vi "UHR-Fleezers Control (host) - 12.2.vi"() -> ()   [LabVIEW 2012] (continued)
            n651 = Wait (ms)(milliseconds to wait=u32 250) -> ()  [unwired: 1 out]
          }
          frame #6 {
            n652 = property on="Start Saving" class="Bool (strict)"("Val(Sgnl)"=TRUE ("Value (Signaling)")) -> ()  [unwired: 2 in, 2 out]
            n653 = Wait (ms)(milliseconds to wait=u32 5000) -> ()  [unwired: 1 out]
          }
          frame #7 {
            w1054 = TRUE ("Value (Signaling)")
            n654 = property on="Rem fb disp offset" class="Bool (strict)"("Val(Sgnl)"=w1054) -> ()  [unwired: 2 in, 2 out]
            n655 = property on="Remove Offset" class="Bool (strict)"("Val(Sgnl)"=w1054) -> ()  [unwired: 2 in, 2 out]
            n656 = Wait (ms)(milliseconds to wait=u32 100) -> ()  [unwired: 1 out]
          }
          frame #8 {
            n657 = case shown="True" w1057 {
              frame False {
              }
              frame True {
                n658 = local write "Trap Trig. Fl."(TRUE ("Value (Signaling)")) -> ()
              }
            }
          }
          frame #9 {
            n659 = case shown="True" "Start dipping after?" {
              frame False {
              }
              frame True {
                n660 = flat-sequence {
                  frame #0 {
                    n661 = Multiply(x="Delay before dipping (s)", y=1000.0) -> (x*y=w1061:dbl)
                    n662 = Wait (ms)(milliseconds to wait=w1061) -> ()  [unwired: 1 out]
                  }
                  frame #1 {
                    n663 = property on="Dip for Protein" class="Bool (strict)"("Val(Sgnl)"=TRUE ("Value (Signaling)")) -> ()  [unwired: 2 in, 2 out]
                    n664 = local write "Scripts"(T1."Dipping" ("Scripts")) -> ()
                  }
                }
              }
            }
          }
        }
      }
      event "Fixed Traps Data\nScript": Value Change {
        n665 = event-data() -> ()  [unwired: 1 in, 5 out]
        n666 = flat-sequence {
          frame #0 {
            n667 = case shown="True" "Green ON" {
              frame False {
              }
              frame True {
                n668 = property on="Green Laser ON/Interlacing" class="Bool (strict)"("Val(Sgnl)"=TRUE) -> ()  [unwired: 2 in, 2 out]
              }
            }
            n669 = local write "Offset (nm)"(0.0 ("Offset (nm)")) -> ()
            n670 = property on="Sample Channel\nFlow" class="Bool (strict)"("Val(Sgnl)"=FALSE ("Value (Signaling)")) -> ()  [unwired: 2 in, 2 out]
            n671 = property on="Trap Delta (MHz)" class="DigNum (strict)"("Val(Sgnl)"="Fixed Traps Trap Delta (MHz)") -> ()  [unwired: 2 in, 2 out]
          }
          frame #1 {
            n672 = Wait (ms)(milliseconds to wait=u32 1000) -> ()  [unwired: 1 out]
          }
          frame #2 {
            n673 = local write "Start Saving"(TRUE ("Start Saving")) -> ()
          }
          frame #3 {
            n674 = local read "Bead Sep. Int. Time (s)"() -> (w1072:dbl)
            n675 = Multiply(x=w1072, y=1000.0) -> (x*y=w1074:dbl)
            n676 = Wait (ms)(milliseconds to wait=w1074) -> ()  [unwired: 1 out]
          }
          frame #4 {
            n677 = property on="Remove Offset" class="Bool (strict)"("Val(Sgnl)"=TRUE ("Value (Signaling)")) -> ()  [unwired: 2 in, 2 out]
          }
          frame #5 {
            n678 = property on="Dip for Protein" class="Bool (strict)"("Val(Sgnl)"="Start dipping after?") -> ()  [unwired: 2 in, 2 out]
          }
        }
      }
      event "Got DNA bead": Value Change {
        n679 = event-data() -> ()  [unwired: 1 in, 5 out]
        n680 = flat-sequence {
          frame #0 {
            n681 = local read "Daq spot flow on"() -> (w1079:bool)
            n682 = case shown="True" w1079 {
              frame False {
              }
              frame True {
                n683 = property on="Sample Channel\nFlow" class="Bool (strict)"("Val(Sgnl)"=TRUE ("Value (Signaling)")) -> ()  [unwired: 2 in, 2 out]
              }
            }
            n684 = property on="Got DNA bead" class="Bool"("Key Focus"=FALSE) -> ()  [unwired: 2 in, 2 out]
          }
          frame #1 {
            n685 = property on="Inject Pump 1" class="Bool (strict)"("Val(Sgnl)"=FALSE ("Value (Signaling)")) -> ()  [unwired: 2 in, 2 out]
          }
          frame #2 {
            n686 = property on="Cal/Data Acq. Spot" class="Bool (strict)"("Val(Sgnl)"=TRUE ("Value (Signaling)")) -> ()  [unwired: 2 in, 2 out]
          }
        }
      }
      event "Take Stepping Data": Value Change {
        n687 = event-data() -> ()  [unwired: 1 in, 5 out]
        n688 = local read "Save ave N"() -> (w1091:dbl)
        n689 = flat-sequence {
          tunnel: w1091 -> [w1093]
          tunnel: [w1093] -> w1086
          tunnel: [w1095] -> w1087
          tunnel: w1086 -> [w1095]
          tunnel: [w1097] -> w1088
          tunnel: w1087 -> [w1097]
          tunnel: [w1100] -> w1089
          tunnel: w1088 -> [w1100]
          tunnel: [w1102] -> w1090
          tunnel: w1089 -> [w1102]
          tunnel: [w1104] -> w1084
          tunnel: w1090 -> [w1104]
          tunnel: w1084 -> [w1107]
          tunnel: [w1107] -> w1083
          tunnel: w1083 -> [w1108]
          tunnel: [w1108] -> w1085
          tunnel: w1085 -> [w1114]
          frame #0 {
            n690 = property on="Save ave N" class="DigNum (strict)"("Val(Sgnl)"="Save ave factor") -> ()  [unwired: 2 in, 2 out]
          }
          frame #1 {
            n691 = Wait (ms)(milliseconds to wait=u32 100) -> ()  [unwired: 1 out]
          }
          frame #2 {
            n692 = local read "Offset 2 Start (MHz)"() -> (w1099:dbl)
            n693 = property on="Saved AOD Raster Scan Parameter Sets" class="Arr (strict)"("Index Values"=u32[] [2]) -> ()  [unwired: 2 in, 2 out]
            n694 = property on="Trap Delta (MHz)" class="DigNum (strict)"("Val(Sgnl)"=w1099) -> ()  [unwired: 2 in, 2 out]
          }
          frame #3 {
            n695 = property on="Load parameters" class="Bool (strict)"("Val(Sgnl)"=TRUE ("Value (Signaling)")) -> ()  [unwired: 2 in, 2 out]
          }
          frame #4 {
            n696 = Wait (ms)(milliseconds to wait=u32 100) -> ()  [unwired: 1 out]
          }
          frame #5 {
            n697 = property on="Trap Raster Scan" class="Bool (strict)"("Val(Sgnl)"=TRUE ("Value (Signaling)")) -> ()  [unwired: 2 in, 2 out]
          }
          frame #6 {
            n698 = Wait (ms)(milliseconds to wait=u32 1000) -> ()  [unwired: 1 out]
          }
          frame #7 {
            n699 = while {
              stop <- w1111 stop-if-true
              n700 = local read "Raster Scanning..."() -> (w1113:bool)
              n701 = local read "Saving..."() -> (w1112:bool)
              n702 = Not(x=w1112) -> (.not. x?=w1109:bool)
              n703 = Not(x=w1113) -> (.not. x?=w1110:bool)
              n704 = And(x=w1110, y=w1109) -> (x .and. y?=w1111:bool)
            }
          }
          frame #8 {
            n705 = property on="Save ave N" class="DigNum (strict)"("Val(Sgnl)"=w1114) -> ()  [unwired: 2 in, 2 out]
          }
        }
      }
      event "Step Size (nm)": Value Change {
        n706 = event-data() -> ()  [unwired: 1 in, 5 out]
        n707 = flat-sequence {
          frame #0 {
            n708 = property on="Saved AOD Raster Scan Parameter Sets" class="Arr (strict)"("Index Values"=u32[] [1]) -> ()  [unwired: 2 in, 2 out]
          }
          frame #1 {
            n709 = Multiply(x="N Steps", y="Step Size (nm)") -> (x*y=w1116:dbl)
            n710 = property on="Scan Speed AOD (nm/s) 2" class="DigNum (strict)"("Value"="Step Size (nm)") -> ()  [unwired: 2 in, 2 out]
            n711 = property on="Step Size AOD (nm) 2" class="DigNum (strict)"("Value"="Step Size (nm)") -> ()  [unwired: 2 in, 2 out]
            n712 = property on="Scan Range AOD (nm) 2" class="DigNum (strict)"("Value"=w1116) -> ()  [unwired: 2 in, 2 out]
          }
        }
      }
      event "Take Detection Laser\nImage": Value Change {
        n713 = event-data() -> ()  [unwired: 1 in, 5 out]
        n714 = flat-sequence {
          tunnel: [w1144] -> w1134
          tunnel: [w1143] -> w1127
          tunnel: [w1142] -> w1119
          tunnel: [w1147] -> w1135
          tunnel: w1134 -> [w1147]
          tunnel: [w1146] -> w1128
          tunnel: w1127 -> [w1146]
          tunnel: [w1145] -> w1120
          tunnel: w1119 -> [w1145]
          tunnel: [w1151] -> w1136
          tunnel: w1135 -> [w1151]
          tunnel: [w1150] -> w1129
          tunnel: w1128 -> [w1150]
          tunnel: [w1149] -> w1121
          tunnel: w1120 -> [w1149]
          tunnel: [w1157] -> w1137
          tunnel: w1136 -> [w1157]
          tunnel: [w1156] -> w1130
          tunnel: w1129 -> [w1156]
          tunnel: [w1155] -> w1122
          tunnel: w1121 -> [w1155]
          tunnel: [w1161] -> w1138
          tunnel: w1137 -> [w1161]
          tunnel: [w1160] -> w1131
          tunnel: w1130 -> [w1160]
          tunnel: [w1159] -> w1123
          tunnel: w1122 -> [w1159]
          tunnel: [w1165] -> w1139
          tunnel: w1138 -> [w1165]
          tunnel: [w1164] -> w1132
          tunnel: w1131 -> [w1164]
          tunnel: [w1163] -> w1124
          tunnel: w1123 -> [w1163]
          tunnel: [w1169] -> w1140
          tunnel: w1139 -> [w1169]
          tunnel: [w1168] -> w1133
          tunnel: w1132 -> [w1168]
          tunnel: [w1167] -> w1125
          tunnel: w1124 -> [w1167]
          tunnel: w1140 -> [w1175]
          tunnel: w1133 -> [w1174]
          tunnel: [w1172] -> w1126
          tunnel: w1125 -> [w1172]
          tunnel: w1126 -> [w1176]
          frame #0 {
            n715 = local read "Green Laser ON/Interlacing"() -> (w1144:bool)
            n716 = local read "Laser interlacing mode"() -> (w1143:enum32{"Laser ON", "Laser OFF", "Interlace"})
            n717 = local read "Green FB On/Off"() -> (w1142:bool)
          }
          frame #1 {
            n718 = property on="Green FB On/Off" class="Bool (strict)"("Val(Sgnl)"=FALSE ("Value (Signaling)")) -> ()  [unwired: 2 in, 2 out]
          }
          frame #2 {
            n719 = property on="Green Laser ON/Interlacing" class="Bool (strict)"("Val(Sgnl)"=TRUE ("Value (Signaling)")) -> ()  [unwired: 2 in, 2 out]
            n720 = property on="Flip Green Filter" class="Bool (strict)"("Val(Sgnl)"=TRUE ("Value (Signaling)")) -> ()  [unwired: 2 in, 2 out]
            n721 = property on="Laser interlacing mode" class="RadioBtnsControl (strict)"("Val(Sgnl)"=enum32{"Laser ON", "Laser OFF", "Interlace"}."Laser ON" ("Value (Signaling)")) -> ()  [unwired: 2 in, 2 out]
          }
          frame #3 {
            n722 = Wait (ms)(milliseconds to wait=u32 500) -> ()  [unwired: 1 out]
          }
          frame #4 {
            n723 = property on="Confocal Image" class="Bool (strict)"("Val(Sgnl)"=TRUE ("Value (Signaling)")) -> ()  [unwired: 2 in, 2 out]
          }
          frame #5 {
            n724 = Wait (ms)(milliseconds to wait=u32 2000) -> ()  [unwired: 1 out]
          }
          frame #6 {
            n725 = while {
              stop <- w1170 stop-if-true
              n726 = local read "Saving..."() -> (w1171:bool)
              n727 = Not(x=w1171) -> (.not. x?=w1170:bool)
            }
          }
          frame #7 {
            n728 = property on="Flip Green Filter" class="Bool (strict)"("Val(Sgnl)"=TRUE ("Value (Signaling)")) -> ()  [unwired: 2 in, 2 out]
            n729 = property on="Green Laser ON/Interlacing" class="Bool (strict)"("Val(Sgnl)"=w1175) -> ()  [unwired: 2 in, 2 out]
            n730 = property on="Laser interlacing mode" class="RadioBtnsControl (strict)"("Val(Sgnl)"=w1174) -> ()  [unwired: 2 in, 2 out]
          }
          frame #8 {
            n731 = property on="Green FB On/Off" class="Bool (strict)"("Val(Sgnl)"=w1176) -> ()  [unwired: 2 in, 2 out]
          }
        }
      }
      event "Stop All": Value Change {
        n732 = event-data() -> ()  [unwired: 1 in, 5 out]
        n733 = local read "Stop All"() -> (w1177:bool)
      }
    }
    n734 = node-c288() -> ()  [unwired: 1 in, 1 out]
  }
  n735 = node-c288(3 ("Processor")) -> (w135:T21)  [unwired: 3 out]
  n736 = flat-sequence "Video" {
    tunnel: [w1187] -> w125
    tunnel: w125 -> [w1227]
    frame #0 {
      n737 = while {
        stop <- w1179 continue-if-true
        n738 = call "Close Video Capture.vi"() -> ("error code OUT"=w1181:i32)
        n739 = Equal?(x=w1181, y=0) -> (x = y?=w1179:bool)
      }
      n740 = local write "Stop All"(FALSE ("Stop All")) -> ()
    }
    frame #1 {
      n741 = call "DMR_Init.vi"() -> ()  [unwired: 3 out]
    }
    frame #2 {
      w1182 = "DE245428202"  # MSU fleezers card #
      (unwired) "DE019116701"  # Illinois fleezers card #
      # "Setting the destination format to Mono8 makes sure that the image can be displayed in the intensity plot."
      n742 = call "DMR_GetDevice.vi"("search string IN"=w1182) -> ("device handle OUT"=w1205:i32)  [unwired: 4 in, 2 out]
      n743 = call "DMR_OpenDevice.vi"("device handle IN"=w1205) -> ("driver handle OUT"=w1188:i32)  [unwired: 4 out]
      n744 = call "DMR_FindList.vi"("flags IN"=u32 0 ("flags"), "list name IN"="" ("String"), "list type IN"=T26."camera descriptions", "driver handle IN"=w1188) -> ("list handle OUT"=w1191:i32)  [unwired: 2 out]
      n745 = call "DMR_FindList.vi"("flags IN"=u32 0 ("flags"), "list name IN"="Base", "list type IN"=T26."setting", "driver handle IN"=w1188) -> ("list handle OUT"=w1189:i32)  [unwired: 2 out]
      n746 = call "OBJ_GetHandle.vi"("object name IN"="VideoStandard", "list handle IN"=w1191) -> ("object handle OUT"=w1185:i32)  [unwired: 3 out]
      n747 = call "OBJ_GetHandle.vi"("object name IN"="PixelFormat", "list handle IN"=w1189) -> ("object handle OUT"=w1199:i32)  [unwired: 3 out]
      n748 = call "OBJ_SetS.vi"("value index IN"=0, "value IN"="NTSC M", "object handle IN"=w1185) -> ()  [unwired: 2 out]
      n749 = call "OBJ_SetS.vi"("value index IN"=0, "value IN"="Mono8" ("value"), "object handle IN"=w1199) -> ()  [unwired: 2 out]
      n750 = call "OBJ_GetHandle.vi"("object name IN"="VideoChannel", "list handle IN"=w1189) -> ("object handle OUT"=w1195:i32)  [unwired: 3 out]
      n751 = while {
        tunnel: [w1209] -> w1187
        tunnel: w1188 -> [w1206]
        stop <- w1207 continue-if-true
        n752 = call "DMR_ImageRequestSingle.vi"("request control IN"=0, "driver handle IN"=w1206) -> ("error code OUT"=w1208:i32, "driver handle OUT"=w1209:i32)  [unwired: 2 out]
        n753 = Equal To 0?(x=w1208) -> (x = 0?=w1207:bool)
      }
      n754 = call "OBJ_SetI.vi"("value index IN"=0, "value IN"=3 ("Video channel"), "object handle IN"=w1195) -> ()  [unwired: 2 out]
    }
    frame #3 {
      w1215 = T17 0 items=["Grayscale (U8)", "Grayscale (I16)", "Grayscale (SGL)", "Complex (CSG)", "RGB (U32)", "HSL (U32)", "RGB (U64)"] ("Image Type")
      w1223 = T17 0 items=["Grayscale (U8)", "Grayscale (I16)", "Grayscale (SGL)", "Complex (CSG)", "RGB (U32)", "HSL (U32)", "RGB (U64)"] ("Image Type")
      n755 = for "Create Greyscale map" {
        N: 256 -> [_]
        tunnel: [w1229] -> w1212 mode=indexing
        workers-P: _ -> [_]
        i -> [w1232]
        n756 = To Unsigned Byte Integer(number=w1232) -> (unsigned 8bit integer=w1228:u8)
        n757 = Join Numbers(hi=w1228, lo=w1228) -> ((hi.lo)=w1231:u16)
        n758 = Join Numbers(hi=w1228, lo=w1228) -> ((hi.lo)=w1230:u16)
        n759 = Join Numbers(hi=w1231, lo=w1230) -> ((hi.lo)=w1229:u32)
      }
      n760 = call "IMAQ Create"("Image Name"="Scaled video", "Image Type"=w1215) -> ("New Image"=w1214:T2)  [unwired: 2 in, 2 out]
      n761 = call "IMAQ Create"("Image Name"="Main video", "Image Type"=w1223) -> ("New Image"=w1224:T2)  [unwired: 2 in, 2 out]
      n762 = node-c288(0 ("Processor")) -> (w1222:T21)  [unwired: 3 out]
      n763 = Initialize Array(u32 0 ("Window Number (0...15)"), 480 ("dimension size"), 640 ("dimension size")) -> (w1217:u32[][])
      n764 = timed-loop {
        tunnel: w1227 -> [w1249]
        tunnel: [w1248] -> w1226
        tunnel: w1224 -> [w1247]
        timing: w1222 -> [_]
        timing-out: [_] -> w1221
        tunnel: w1217 -> [w1236]
        tunnel: w1214 -> [w1234]
        tunnel: w1212 -> [w1233]
        stop <- w1235 stop-if-true
        # "This block performs the \nactual image capture."
        n765 = node-c288() -> ()  [unwired: 2 out]
        n766 = local read "Stop All"() -> (w1235:bool)
        n767 = Reciprocal(x="Video Capture Rate (Hz)") -> (1/x=w1239:dbl)
        n768 = Multiply(x=w1239, y=1000.0) -> (x*y=w1237:dbl)
        n769 = call "DMR_ImageRequestWaitFor.vi"("queue number IN"=0, "timeout(ms) IN"=500, "driver handle IN"=w1249) -> ("error code OUT"=w1253:i32, "request number OUT"=w1250:i32, "driver handle OUT"=w1251:i32)
        n770 = feedback #1(T27 refnum ("Avi Refnum")) -> (w1241:T27)
        n771 = case shown="True" "New Video File" {
          tunnel: [T27 refnum ("Avi Refnum") w1270] -> w1243
          tunnel: [FALSE TRUE] -> w1244
          tunnel: w1241 -> [_ w1266]
          frame False {
          }
          frame True {
            n772 = call "Create new save file.vi"("Ext"=".avi" ("string"), "Index In"="Video Index") -> ("Path Out"=w1262:path, "Index Out"=w1263:dbl)  [unwired: 1 in]
            "Path Out" <- w1262
            n773 = Not Equal?(x=w1266, y=T27 refnum ("Avi Refnum")) -> (x != y?=w1267:bool)
            n774 = Increment(x=w1263) -> (x+1=w1272:dbl)
            n775 = case shown="True" w1267 {
              tunnel: w1266 -> [_ w1273]
              frame False {
              }
              frame True {
                n776 = call "IMAQ AVI Close"("Avi Refnum"=w1273) -> ()  [unwired: 1 in, 10 out]
              }
            }
            n777 = local write "Video Index"(w1272) -> ()
            n778 = call "IMAQ AVI Create"("Frames Per Second"=u32 30, "AVI Path"=w1262) -> ("Avi Refnum"=w1270:T27)  [unwired: 5 in, 4 out]
          }
        }
        n779 = Equal To 0?(x=w1253) -> (x = 0?=w1252:bool)
        n780 = Select(t=w1243, s=w1244, f=w1241) -> (s? t:f=w1242:T27)
        n781 = feedback-in #1(w1242) -> ()
        n782 = case shown="True" w1252 {
          tunnel: w1251 -> [w1274 w1299]
          tunnel: w1250 -> [_ w1298]
          tunnel: [w1274 w1295] -> w1248
          tunnel: w1247 -> [_ w1279]
          tunnel: w1236 -> [_ w1283]
          tunnel: w1242 -> [_ w1281]
          tunnel: w1234 -> [_ w1276]
          tunnel: w1233 -> [_ w1275]
          frame False {
          }
          frame True {
            w1289 = u32 0 ("X-offset IN")
            n783 = call "DMR_GetImageRequestBufferData.vi"("driver handle IN"=w1299, "request number IN"=w1298) -> ("width OUT"=w1288:i32, "height OUT"=w1287:i32, "driver handle OUT"=w1294:i32, "request number OUT"=w1293:i32, "bytes per pixel OUT"=w1290:i32)  [unwired: 13 out]
            n784 = call "DMR_GetImageRequestBufferImageData.vi"("driver handle IN"=w1294, "request number IN"=w1293, "bytes per pixel IN"=w1290, "X-offset IN"=w1289, "Y-offset IN"=w1289, "height IN"=w1287, "width IN"=w1288) -> ("driver handle OUT"=w1292:u32, "request number OUT"=w1291:u32, "image OUT"=w1284:u32[][])  [unwired: 10 out]
            n785 = call "DMR_ImageRequestUnlock.vi"("request number IN"=w1291, "driver handle IN"=w1292) -> ("driver handle OUT"=w1297:i32)  [unwired: 1 in, 2 out]
            n786 = case shown="True" "Averaging" {
              tunnel: w1284 -> [w1335 w1340]
              tunnel: [w1335 w1339] -> w1280
              tunnel: w1283 -> [_ w1337]
              frame False {
              }
              frame True {
                (unwired) 1
                w1345 = 1
                n787 = feedback #2(w1337) -> (w1336:u32[][])
                n788 = Add(x=w1340, y=w1336) -> (x+y=w1341:u32[][])
                n789 = Select(t=w1337, s="Reset Averaging", f=w1341) -> (s? t:f=w1343:u32[][])
                n790 = feedback-in #2(w1343) -> ()
                n791 = feedback #3(w1345) -> (w1338:i32)
                n792 = Divide(x=w1341, y=w1338) -> (x/y=w1342:dbl[][])
                n793 = Increment(x=w1338) -> (x+1=w1346:i32)
                n794 = To Unsigned Long Integer(number=w1342) -> (unsigned 32bit integer=w1339:u32[][])
                n795 = Select(t=w1345, s="Reset Averaging", f=w1346) -> (s? t:f=w1344:i32)
                n796 = feedback-in #3(w1344) -> ()
              }
            }
            n797 = call "DMR_ImageRequestSingle.vi"("request control IN"=0, "driver handle IN"=w1297) -> ("driver handle OUT"=w1295:i32)  [unwired: 3 out]
            n798 = disable-structure shown="Disabled" {
              disable-tunnel: w1280 -> [w1312 _]
              disable-tunnel: w1276 -> [w1311 _]
              frame Disabled {
                n799 = To Double Precision Float(number=w1312) -> (double precision float=w1310:dbl[][])
                n800 = In Range and Coerce(upper limit="Intensity Upper", x=w1310, lower limit="Intensity Lower") -> (coerced(x)=w1309:dbl[][])  [unwired: 1 out]
                n801 = Subtract(x="Intensity Upper", y="Intensity Lower") -> (x-y=w1306:dbl)
                n802 = Subtract(x=w1309, y="Intensity Lower") -> (x-y=w1307:dbl[][])
                n803 = Divide(x=w1307, y=w1306) -> (x/y=w1308:dbl[][])
                n804 = Multiply(x=255.0, y=w1308) -> (x*y=w1304:dbl[][])
                n805 = To Unsigned Byte Integer(number=w1304) -> (unsigned 8bit integer=w1313:u8[][])
                n806 = call "IMAQ ArrayToImage"("Image Pixels (U8)"=w1313, "Image"=w1311) -> ("Image Out"=w1300:T2)  [unwired: 4 in, 5 out]
                n807 = First Call?() -> (First Call?: T/F=w1301:bool)
                n808 = case shown="True" w1301 {
                  tunnel: w1300 -> [w1314 w1325]
                  frame False {
                    n809 = flat-sequence {
                      tunnel: w1314 -> [w1320]
                      frame #0 {
                        w1317 = FALSE ("Get/Set Status? (Set)")
                        w1316 = 0 ("Window Number (0...15)")
                        n810 = call "IMAQ WindSize"("Get/Set Status? (Set)"=w1317, "Window Number"=w1316) -> ("Width & Height out"=→"Window Size":cluster{"Width":i32, "Height":i32})  [unwired: 4 in, 2 out]
                        n811 = call "IMAQ WindMove"("Window Number (0...15)"=w1316, "Get/Set Status? (Set)"=w1317) -> ("Coordinates (screen)"=→"Window Position":cluster{"X Position":i32, "Y Position":i32})  [unwired: 3 in, 1 out]
                        n812 = call "IMAQ WindDraw"("Resize to Image Size? (Y)"=FALSE, "Window Number (0...15)"=w1316, "Image"=w1320) -> ()  [unwired: 7 in, 2 out]
                      }
                      frame #1 {
                        n813 = call "IMAQ WindZoom 2"("Center Point"="Center Point", "Zoom to Fit? (False)"=FALSE, "Zoom Factor"="Zoom Factor") -> ()  [unwired: 5 in, 4 out]
                      }
                    }
                  }
                  frame True {
                    n814 = flat-sequence {
                      tunnel: w1325 -> [w1328]
                      tunnel: [w1326] -> w1324
                      tunnel: w1324 -> [w1330]
                      frame #0 {
                        w1327 = TRUE ("Resize to Image Size? (Y)")
                        w1326 = 0 ("Window Number (0...15)")
                        n815 = call "IMAQ WindNonTearing"("Window Number"=w1326, "NonTearing? (True)"=w1327) -> ()  [unwired: 8 in, 2 out]
                        n816 = call "IMAQ WindDraw"("Resize to Image Size? (Y)"=w1327, "Window Number (0...15)"=w1326, "Image"=w1328) -> ()  [unwired: 7 in, 2 out]
                      }
                      frame #1 {
                        n817 = call "IMAQ WindSize"("Scrollbars? (N)"=FALSE, "Width & Height"="Initial Window Size", "Window Number"=w1330) -> ()  [unwired: 3 in, 3 out]
                        n818 = call "IMAQ WindMove"("Window Number (0...15)"=w1330, "Coordinates (screen)"="Initial Window Position") -> ()  [unwired: 3 in, 2 out]
                      }
                    }
                  }
                }
              }
              frame Enabled {
              }
            }
            n819 = To Unsigned Byte Integer(number=w1280) -> (unsigned 8bit integer=w1278:u8[][])
            n820 = call "IMAQ ArrayToImage"("Image Pixels (U8)"=w1278, "Image"=w1279) -> ("Image Out"=w1277:T2)  [unwired: 4 in, 5 out]
            "Primary Video Display" <- w1277
            n821 = case shown="True" "Save Video" {
              tunnel: w1281 -> [_ w1334]
              tunnel: w1277 -> [_ w1333]
              frame False {
              }
              frame True {
                n822 = call "IMAQ AVI Write Frame"("Image"=w1333, "Avi Refnum"=w1334) -> ()  [unwired: 2 in, 8 out]
              }
            }
            n823 = case shown="True" "Save Image" {
              tunnel: w1278 -> [_ w1349]
              tunnel: w1275 -> [_ w1348]
              frame False {
              }
              frame True {
                n824 = call <vilib>:"Flatten Pixmap.vi"("colors"=w1348, "8-bit pixmap"=w1349) -> ("image data"=w1355:T28)  [unwired: 4 in, 5 out]
                n825 = call "Create new save file.vi"("Insert"="video_frame_" ("string"), "Ext"=".bmp" ("string"), "Index In"="Image Index") -> ("Path Out"=w1351:path, "Index Out"=w1356:dbl)
                n826 = Increment(x=w1356) -> (x+1=w1350:dbl)
                n827 = local write "Image Index"(w1350) -> ()
                n828 = call <vilib>:"Write BMP File.vi"("image data"=w1355, "path to BMP file"=w1351) -> ()  [unwired: 1 in, 9 out]
              }
            }
          }
        }
        n829 = node-c288(w1237) -> ()  [unwired: 1 out]
      }
      n830 = node-c288(w1221) -> ()  [unwired: 1 out]
      n831 = call "DMR_CloseDevice.vi"("driver handle IN"=w1226) -> ()  [unwired: 1 in, 4 out]
    }
    frame #4 {
      n832 = call "DMR_Close.vi"() -> ()  [unwired: 1 out]
    }
  }
  n833 = timed-loop "Acquire Data" {
    tunnel: w52 -> [w1652]
    tunnel: w97 -> [w1651]
    tunnel: [w1681] -> w305
    tunnel: [w1676] -> w303
    timing: w213 -> [_]
    timing-out: [_] -> w212
    tunnel: w114 -> [w1497]
    stop <- "Stop All" stop-if-true
    w1412 = "Initialize"
    w1482 = "NI_ChannelName" ("name")
    n834 = node-c288() -> ()  [unwired: 2 out]
    n835 = First Call?() -> (First Call?: T/F=w1447:bool)
    n836 = Or(x="Reset", y=w1447) -> (x .or. y?=w1448:bool)
    n837 = local read "Flushing P1"() -> (w1367:bool)
    n838 = case "Reset data stream" shown="True" w1448 {
      tunnel: w1652 -> [w2669 w2677]
      tunnel: w1651 -> [w2668 w2676]
      tunnel: [w2669 w2671] -> w1647
      tunnel: [w2668 w2670] -> w1646
      frame False {
      }
      frame True {
        w2674 = TRUE ("AI to FIFO")
        n839 = local write "Overflow (data lost)"(FALSE ("Overflow (data lost)")) -> ()
        n840 = call "reset FPGA DMA.vi"("error in"=w2676, "FPGA VI Reference In"=w2677) -> ("error out"=w2672:errorcluster, "FPGA VI Reference Out"=w2673:T19)
        n841 = xnode "Read/Write Control"("FPGA VI Reference In"=w2673, "error in"=w2672, "AI to FIFO"=w2674, "APD to FIFO"=w2674) -> ("FPGA VI Reference Out"=w2671:T19, "error out"=w2670:errorcluster)
      }
    }
    n842 = case shown="True" w1367 {
      frame False {
      }
      frame True {
        n843 = local read "Flush rate (uL/m) P1"() -> (w1698:dbl)
        n844 = local read "HP1 Flush Time (s)"() -> (w1707:dbl)
        n845 = local read "DMA Update Period (s)"() -> (w1701:dbl)
        n846 = Divide(x=w1698, y=60.0) -> (x/y=w1699:dbl)
        n847 = Divide(x=w1707, y=w1701) -> (x/y=w1696:dbl)
        n848 = feedback #4(0) -> (w1705:i32)
        n849 = Increment(x=w1705) -> (x+1=w1695:i32)
        n850 = Greater?(x=w1695, y=w1696) -> (0:w1704:bool)
        n851 = Compound Arithmetic op=MULTIPLY(w1701, w1695, w1699) -> (→"P1 Flush Volume (uL)":dbl)
        n852 = Divide(x=w1695, y=w1696) -> (x/y=→"P1 Flushing Bar":dbl)
        n853 = case shown="True" w1704 {
          tunnel: w1695 -> [w1708 _]
          tunnel: [w1708 0] -> w1703
          frame False {
          }
          frame True {
            w1709 = FALSE ("Flushing P1")
            n854 = local write "Inject Pump 1"(w1709) -> ()
            n855 = local write "Flushing P1"(w1709) -> ()
            n856 = property on="Clear Volume P1" class="Bool (strict)"("Val(Sgnl)"=TRUE ("Value (Signaling)")) -> ()  [unwired: 2 in, 2 out]
          }
        }
        n857 = feedback-in #4(w1703) -> ()
      }
    }
    n858 = Or(x="Start AOD Scan", y="Trap Raster Scan") -> (x .or. y?=w1603:bool)
    n859 = case "Start AOM raster scan" shown="True" w1603 {
      tunnel: w1647 -> [w2519 w2529]
      tunnel: w1646 -> [w2518 w2528]
      tunnel: [w2519 w2522] -> w1645
      tunnel: [w2518 w2521] -> w1644
      frame False {
      }
      frame True {
        n860 = case shown="True" "Restart DMA? (AOD)" {
          tunnel: [w2567 w2569] -> w2523
          tunnel: [w2566 w2568] -> w2524
          tunnel: w2529 -> [w2567 w2571]
          tunnel: w2528 -> [w2566 w2570]
          frame False {
          }
          frame True {
            n861 = local write "Overflow (data lost)"(FALSE ("Overflow (data lost)")) -> ()
            n862 = call "reset FPGA DMA.vi"("error in"=w2570, "FPGA VI Reference In"=w2571) -> ("error out"=w2568:errorcluster, "FPGA VI Reference Out"=w2569:T19)
          }
        }
        n863 = local write "Trap Raster Scan"(FALSE ("Trap Raster Scan")) -> ()
        n864 = case shown="True" "Move MCL Also?" {
          tunnel: w2524 -> [w2532 w2561]
          tunnel: w2523 -> [w2533 w2562]
          tunnel: [w2531 w2565] -> w2522
          tunnel: [w2530 w2564] -> w2521
          frame False {
            w2534 = TRUE ("AI to FIFO")
            n865 = xnode "Read/Write Control"("FPGA VI Reference In"=w2533, "error in"=w2532, "AI to FIFO"=w2534, "APD to FIFO"=w2534, "Start scan"=w2534) -> ("FPGA VI Reference Out"=w2531:T19, "error out"=w2530:errorcluster)
          }
          frame True {
            w2558 = FALSE ("1D or 2D Scan?")
            w2563 = TRUE ("AI to FIFO")
            # "Count for MCL loop"
            # "N total cycles"
            # "N steps"
            # "V_int"
            n866 = local read "Scan Range (nm)"() -> (w2540:dbl)
            n867 = local read "Number of F/B Scans (AOD)"() -> (w2557:u16)
            n868 = Sign(1:w2540) -> (0:w2539:dbl)
            n869 = Compound Arithmetic op=MULTIPLY(w2540, "MCL Step Position Ratio", "MCL/AOM Scale Tweak") -> (w2544:dbl)
            n870 = Negate(x=w2539) -> (-x=w2536:dbl)
            n871 = Multiply(x=w2536, y="MCL Step Increment (V_int)") -> (x*y=w2538:dbl)
            n872 = Divide(x=w2544, y="MCL X Cal (nm/V)") -> (x/y=w2550:dbl)
            n873 = Multiply(x=32767.0 ("y"), y=w2550) -> (x*y=w2556:dbl)
            n874 = local read "Total Counts (ticks)"() -> (w2541:u32)
            n875 = local read "Cycles/step (AOD)"() -> (w2552:u64)
            n876 = local read "Scan steps (AOD)"() -> (w2553:u64)
            n877 = Divide(x=w2556, y=10.0) -> (x/y=w2549:dbl)
            n878 = Divide(x=w2549, y="MCL Step Increment (V_int)") -> (x/y=w2547:dbl)
            n879 = Absolute Value(x=w2547) -> (abs(x)=w2535:dbl)
            n880 = Compound Arithmetic op=MULTIPLY(w2553, w2552, w2541) -> (w2548:u64)
            n881 = local write "wait to reset values"(w2563) -> ()
            n882 = local write "MCL Scanning"(w2563) -> ()
            n883 = Divide(x=w2548, y=w2535) -> (x/y=w2545:dbl)
            "MCL Count" <- w2545
            n884 = xnode "Read/Write Control"("FPGA VI Reference In"=w2562, "error in"=w2561, "Scan steps (MCL)"=w2535, "Number of scans (MCL)"=w2557, "Cycles per step (MCL)"=u64 1, "Scan freq.  increment (MCL)"=w2538, "1D or 2D Scan?"=w2558, "MCL Scan Axis"=w2558, "Cont. Scan (MCL)"=w2558, "MCL count"=w2545) -> ("FPGA VI Reference Out"=w2560:T19, "error out"=w2559:errorcluster)
            n885 = xnode "Read/Write Control"("FPGA VI Reference In"=w2560, "error in"=w2559, "AI to FIFO"=w2563, "APD to FIFO"=w2563, "Start scan"=w2563, "Start scan (MCL)"=w2563) -> ("FPGA VI Reference Out"=w2565:T19, "error out"=w2564:errorcluster)
          }
        }
        "Raster Scanning..." <- TRUE ("Scanning...")
      }
    }
    n886 = local read "Flushing P3"() -> (w1368:bool)
    n887 = case "Keep track of when Harvard Pump 3 is done flushing" shown="True" w1368 {
      frame False {
      }
      frame True {
        n888 = local read "Flush rate (uL/m) P3"() -> (w1715:dbl)
        n889 = local read "DMA Update Period (s)"() -> (w1717:dbl)
        n890 = local read "HP3 Flush Time (s)"() -> (w1724:dbl)
        n891 = Divide(x=w1715, y=60.0) -> (x/y=w1713:dbl)
        n892 = feedback #5(0) -> (w1722:i32)
        n893 = Increment(x=w1722) -> (x+1=w1716:i32)
        n894 = Divide(x=w1724, y=w1717) -> (x/y=w1718:dbl)
        n895 = Greater?(x=w1716, y=w1718) -> (0:w1721:bool)
        n896 = Compound Arithmetic op=MULTIPLY(w1717, w1716, w1713) -> (→"P3 Flush Volume (uL)":dbl)
        n897 = case shown="True" w1721 {
          tunnel: w1716 -> [w1725 _]
          tunnel: [w1725 0] -> w1720
          frame False {
          }
          frame True {
            w1726 = FALSE ("Flushing P3")
            n898 = local write "Inject Pump 3"(w1726) -> ()
            n899 = local write "Flushing P3"(w1726) -> ()
            n900 = property on="Clear Volume P3" class="Bool (strict)"("Val(Sgnl)"=TRUE ("Value (Signaling)")) -> ()  [unwired: 2 in, 2 out]
          }
        }
        n901 = feedback-in #5(w1720) -> ()
        n902 = Divide(x=w1716, y=w1718) -> (x/y=→"P3 Flushing Bar":dbl)
      }
    }
    n903 = And(x="Save scans", y=w1603) -> (x .and. y?=w1643:bool)
    n904 = Compound Arithmetic op=OR("Start MCL Scan", "Confocal Image", "Confocal Linescan") -> (w1601:bool)
    n905 = And(x="Save Data (MCL)", y=w1601) -> (x .and. y?=w1642:bool)
    n906 = case "Start MCL raster scan" shown="True" w1601 {
      tunnel: w1645 -> [w2131 w2147]
      tunnel: w1644 -> [w2130 w2146]
      tunnel: [w2131 w2142] -> w1495
      tunnel: [w2130 w2141] -> w1494
      tunnel: [FALSE w2140] -> w1628
      tunnel: "Start MCL Scan" -> [_ w2135]
      tunnel: "Confocal Image" -> [_ w2134]
      tunnel: "Confocal Linescan" -> [_ _]
      frame False {
      }
      frame True {
        w2140 = TRUE
        n907 = case shown="True" "Restart DMA? (MCL)" {
          tunnel: [w2192 w2194] -> w2145
          tunnel: [w2191 w2193] -> w2144
          tunnel: w2147 -> [w2192 w2197]
          tunnel: w2146 -> [w2191 w2196]
          frame False {
          }
          frame True {
            n908 = call "reset FPGA DMA.vi"("error in"=w2196, "FPGA VI Reference In"=w2197) -> ("error out"=w2193:errorcluster, "FPGA VI Reference Out"=w2194:T19)
            n909 = local write "Overflow (data lost)"(FALSE ("Overflow (data lost)")) -> ()
          }
        }
        n910 = case shown="False" w2135 {
          selector: w2135 -> [_ w2151]
          tunnel: w2134 -> [w2150 _]
          tunnel: [w2150 w2151] -> w2133
          frame False {
            n911 = property on="2D or 1D Scan" class="Bool (strict)"("Val(Sgnl)"=w2150) -> ()  [unwired: 2 in, 2 out]
            n912 = property on="Confocal Image" class="Bool (strict)"("Value"=FALSE ("Start Confocal Map")) -> ()  [unwired: 2 in, 2 out]
          }
          frame True {
          }
        }
        n913 = local write "MCL Scanning"(w2140) -> ()
        n914 = local read "AO1"() -> (w2137:dbl)
        n915 = local read "AO2"() -> (w2136:dbl)
        n916 = case shown="True" "Center Scan" {
          tunnel: w2145 -> [w2158 w2190]
          tunnel: w2144 -> [w2157 w2189]
          tunnel: [w2156 w2188] -> w2142
          tunnel: [w2155 w2187] -> w2141
          tunnel: [w2153 w2174] -> w2139
          tunnel: [w2152 w2173] -> w2138
          tunnel: w2137 -> [w2153 w2179]
          tunnel: w2136 -> [w2152 w2182]
          tunnel: w2133 -> [_ _]
          frame False {
            w2154 = TRUE ("AI to FIFO")
            n917 = xnode "Read/Write Control"("FPGA VI Reference In"=w2158, "error in"=w2157, "AI to FIFO"=w2154, "APD to FIFO"=w2154, "Start scan (MCL)"=w2154) -> ("FPGA VI Reference Out"=w2156:T19, "error out"=w2155:errorcluster)
          }
          frame True {
            w2186 = TRUE ("AI to FIFO")
            n918 = local read "Scan steps (MCL)"() -> (w2165:u64)
            n919 = local read "Scan lines (y)"() -> (w2161:u64)
            n920 = local read "Fast Scan Dir"() -> (w2172:bool)
            n921 = local read "Actual MCL Inc (V)"() -> (w2162:dbl)
            n922 = Decrement(x=w2161) -> (x-1=w2160:u64)
            n923 = Decrement(x=w2165) -> (x-1=w2164:u64)
            n924 = Multiply(x=w2162, y=w2160) -> (x*y=w2159:dbl)
            n925 = Divide(x=w2159, y=2.0) -> (x/y=w2169:dbl)
            n926 = Multiply(x=w2162, y=w2164) -> (x*y=w2163:dbl)
            n927 = Divide(x=w2163, y=2.0) -> (x/y=w2168:dbl)
            n928 = Select(t=w2168, s=w2172, f=w2169) -> (s? t:f=w2167:dbl)
            n929 = Select(t=w2169, s=w2172, f=w2168) -> (s? t:f=w2171:dbl)
            n930 = Subtract(x=w2179, y=w2171) -> (x-y=w2170:dbl)
            n931 = Subtract(x=w2182, y=w2167) -> (x-y=w2166:dbl)
            n932 = local read "2D or 1D Scan"() -> (w2184:bool)
            n933 = Not(x=w2172) -> (.not. x?=w2178:bool)
            n934 = Not(x=w2184) -> (.not. x?=w2180:bool)
            n935 = And(x=w2172, y=w2180) -> (x .and. y?=w2181:bool)
            n936 = And(x=w2180, y=w2178) -> (x .and. y?=w2183:bool)
            n937 = Select(t=w2182, s=w2183, f=w2166) -> (s? t:f=w2173:dbl)
            n938 = Select(t=w2179, s=w2181, f=w2170) -> (s? t:f=w2174:dbl)
            n939 = call "Volt to I16.vi"("Voltage In"=w2174) -> ("I16 Voltage Out"=w2177:i16)
            n940 = call "Volt to I16.vi"("Voltage In"=w2173) -> ("I16 Voltage Out"=w2176:i16)
            n941 = xnode "Read/Write Control"("FPGA VI Reference In"=w2190, "error in"=w2189, "AI to FIFO"=w2186, "APD to FIFO"=w2186, "Start scan (MCL)"=w2186, "AO1"=w2177, "AO2"=w2176) -> ("FPGA VI Reference Out"=w2188:T19, "error out"=w2187:errorcluster)
          }
        }
        "Initial Y" <- w2139
        "Initial X" <- w2138
        n942 = local write "Tab Control 6"(T3."Imaging" ("Tab Control 6")) -> ()
        "wait to reset values" <- w2140
      }
    }
    n943 = local read "Trap Pos Elements/DMA read"() -> (w1491:u32)
    n944 = local read "Trap AI Elements/DMA read"() -> (w1566:u32)
    n945 = local read "APD Elements/DMA read"() -> (w1532:u32)
    n946 = xnode "Get APD Data"("FPGA VI Reference In"=w1495, "error in"=w1494, "Number of Elements"=w1532, "Timeout (ms)"=-1) -> ("Data"=w1531:u32[], "Elements Remaining"=→"APD FIFO Elements Remaining":u32)  [unwired: 2 out]
    n947 = xnode "Invoke Method"("FPGA VI Reference In"=w1495, "error in"=w1494, "Number of Elements"=w1491, "Timeout (ms)"=-1) -> ("Data"=w1454:u16[], "Elements Remaining"=→"Trap Pos FIFO El Remaining":u32)  [unwired: 2 out]
    n948 = xnode "Get Trap Data"("FPGA VI Reference In"=w1495, "error in"=w1494, "Number of Elements"=w1566, "Timeout (ms)"=-1 ("Timeout")) -> ("FPGA VI Reference Out"=w1389:T19, "error out"=w1388:errorcluster, "Data"=w1455:i16[], "Elements Remaining"=w1689:u32)
    "FIFO El. Rem." <- w1689
    n949 = local read "Trap AI FIFO Depth"() -> (w1691:u32)
    n950 = Subtract(x=w1691, y=w1566) -> (x-y=w1690:u32)
    n951 = Decimate 1D Array(w1454) -> (w1451:u16[], w1453:u16[], w1452:u16[])
    n952 = Divide(x=w1689, y=w1690) -> (x/y=w1688:dbl)
    "Buffer Status" <- w1688
    n953 = To Unsigned Long Integer(number=w1451) -> (unsigned 32bit integer=w1450:u32[])
    n954 = Join Numbers(hi=w1453, lo=w1452) -> ((hi.lo)=w1449:u32[])
    n955 = Equal?(x=w1688, y=1.0) -> (x = y?=w1686:bool)
    n956 = Join Numbers(hi=w1450, lo=w1449) -> ((hi.lo)=w1443:u64[])
    n957 = call "IR AOM word to freq - vec.vi"("Frequency Word In (double vec)"=w1443) -> ("Frequency Out"=w1490:dbl[])
    n958 = case "Alert buffer overflow" shown="True" w1686 {
      frame False {
      }
      frame True {
        n959 = call <vilib>:"Beep.vi"() -> ()  [unwired: 3 in, 9 out]
        "Overflow (data lost)" <- TRUE ("Overflow (data lost)")
      }
    }
    n960 = Decimate 1D Array(w1490) -> (w1489:dbl[], w1488:dbl[])
    n961 = Build Array(w1489, w1488) -> (w1487:dbl[][])
    n962 = local read "Trap Sets"() -> (w1565:u32)
    n963 = case "Deinterlace trap data, average down PSD" shown="2" w1565 {
      tunnel: w1455 -> [w2227 w2292]
      tunnel: [w2224 w2289] -> w1558
      tunnel: [w2227 w2291] -> w1446
      tunnel: "Detector Type" -> [w2226 w2287]
      tunnel: [w2225 w2290] -> w1557
      tunnel: [w2223 w2288] -> w1663
      frame 1, Default {
        n964 = Divide(x=w2227, y=3276.7) -> (x/y=w2228:dbl[])
        n965 = Decimate 1D Array(w2228) -> (w2237:dbl[], w2236:dbl[], w2235:dbl[], w2234:dbl[], w2233:dbl[], w2232:dbl[], w2231:dbl[], w2230:dbl[])
        n966 = case shown="\"IR-QPD + PSD + FB-QPD position\"" w2226 {
          tunnel: w2237 -> [w2261 w2286]
          tunnel: w2236 -> [w2260 w2285]
          tunnel: w2235 -> [w2245 w2263]
          tunnel: w2234 -> [w2246 w2273]
          tunnel: w2233 -> [w2259 w2284]
          tunnel: w2232 -> [w2258 w2283]
          tunnel: w2231 -> [w2242 w2264]
          tunnel: w2230 -> [w2241 w2262]
          tunnel: [w2240 w2270] -> w2225
          tunnel: [w2239 w2269] -> w2224
          tunnel: [w2238 w2268] -> w2223
          frame "IR-QPD + PSD + FB-QPD", Default {
            w2238 = 0  # Channel pattern
            n967 = Divide(x=w2261, y=w2246) -> (x/y=w2248:dbl[])
            n968 = Divide(x=w2260, y=w2246) -> (x/y=w2247:dbl[])
            n969 = Divide(x=w2259, y=w2242) -> (x/y=w2244:dbl[])
            n970 = Divide(x=w2258, y=w2241) -> (x/y=w2243:dbl[])
            n971 = Build Array(w2248, w2247, w2246, w2245, w2244, w2243, w2242, w2241) -> (w2239:dbl[][])
            n972 = Bundle("T1 Y", "T1 X", "T1 Sum", "FB Sum", "PSD Y", "PSD X", "PSD Y Sum", "PSD X Sum") -> (w2257:T37)  [unwired: 1 out]
            n973 = Cluster To Array(cluster=w2257) -> (array=w2240:string[])
          }
          frame "IR-QPD + PSD + FB-QPD position" {
            w2268 = 3  # Channel pattern
            n974 = Negate(x=w2264) -> (-x=w2265:dbl[])
            n975 = Divide(x=w2286, y=w2273) -> (x/y=w2275:dbl[])
            n976 = Divide(x=w2285, y=w2273) -> (x/y=w2274:dbl[])
            n977 = Divide(x=w2284, y=w2264) -> (x/y=w2272:dbl[])
            n978 = Divide(x=w2283, y=w2265) -> (x/y=w2271:dbl[])
            n979 = Build Array(w2275, w2274, w2273, w2262, w2263, w2272, w2271, w2264) -> (w2269:dbl[][])
            n980 = Bundle("T1 Y", "T1 X", "T1 Sum", "FB X", "FB Sum", "PSD Y", "PSD X", "PSD Y Sum") -> (w2282:T37)  [unwired: 1 out]
            n981 = Cluster To Array(cluster=w2282) -> (array=w2270:string[])
          }
        }
      }
      frame 2 {
        n982 = case shown="\"IR-QPD + PSD + FB-QPD X position\"" w2287 {
          tunnel: w2292 -> [w2354 w2426 w2497]
          tunnel: [w2293 w2417 w2428] -> w2291
          tunnel: [w2320 w2408 w2475] -> w2290
          tunnel: [w2319 w2371 w2442] -> w2289
          tunnel: [w2313 w2406 w2473] -> w2288
          frame "IR-QPD + PSD + FB-QPD", Default {
            w2313 = 1  # Channel pattern
            # "time average x2 the 4th signal and the 4 psd signals (detection laser)"
            # "deinterlace 3 signals from qpd"
            n983 = Decimate 1D Array(w2354) -> (w2353:i16[], w2352:i16[], w2318:i16[], w2351:i16[], w2341:i16[], w2339:i16[], w2338:i16[], w2336:i16[])
            n984 = Decimate 1D Array(w2318) -> (w2317:i16[], w2316:i16[])
            n985 = Decimate 1D Array(w2353) -> (w2350:i16[], w2322:i16[])
            n986 = Decimate 1D Array(w2352) -> (w2349:i16[], w2347:i16[])
            n987 = Decimate 1D Array(w2351) -> (w2348:i16[], w2346:i16[])
            n988 = call "downsample 1D array - double.vi"("Ave N"=2.0, "Array In"=w2341) -> ("Array Out"=w2340:dbl[])  [unwired: 1 out]
            n989 = call "downsample 1D array - double.vi"("Ave N"=2.0, "Array In"=w2339) -> ("Array Out"=w2321:dbl[])  [unwired: 1 out]
            n990 = call "downsample 1D array - double.vi"("Ave N"=2.0, "Array In"=w2338) -> ("Array Out"=w2337:dbl[])  [unwired: 1 out]
            n991 = call "downsample 1D array - double.vi"("Ave N"=2.0, "Array In"=w2336) -> ("Array Out"=w2335:dbl[])  [unwired: 1 out]
            n992 = Interleave 1D Arrays(w2350, w2349, w2348, w2322, w2347, w2346, w2317, w2316, w2340, w2321, w2337, w2335) -> (w2334:dbl[])
            n993 = Divide(x=w2334, y=3276.7) -> (x/y=w2333:dbl[])
            n994 = Decimate 1D Array(w2333) -> (w2332:dbl[], w2331:dbl[], w2330:dbl[], w2329:dbl[], w2328:dbl[], w2327:dbl[], w2315:dbl[], w2314:dbl[], w2326:dbl[], w2325:dbl[], w2324:dbl[], w2323:dbl[])
            n995 = Divide(x=w2332, y=w2330) -> (x/y=w2300:dbl[])
            n996 = Divide(x=w2331, y=w2330) -> (x/y=w2299:dbl[])
            n997 = Divide(x=w2329, y=w2327) -> (x/y=w2298:dbl[])
            n998 = Divide(x=w2328, y=w2327) -> (x/y=w2297:dbl[])
            n999 = Divide(x=w2326, y=w2324) -> (x/y=w2296:dbl[])
            n1000 = Divide(x=w2325, y=w2323) -> (x/y=w2295:dbl[])
            n1001 = Build Array(w2300, w2299, w2330, w2298, w2297, w2327, w2315, w2314, w2296, w2295, w2324, w2323) -> (w2319:dbl[][])
            n1002 = Bundle("T1 Y", "T1 X", "T1 Sum", "T2 Y", "T2 X", "T2 Sum", "T1 FB Sum", "T2 FB Sum", "PSD Y", "PSD X", "PSD Y Sum", "PSD X Sum") -> (w2301:T38)  [unwired: 1 out]
            n1003 = To Word Integer(number=w2334) -> (16bit integer=w2293:i16[])
            n1004 = Cluster To Array(cluster=w2301) -> (array=w2320:string[])
          }
          frame "IR-QPD + PSD + FB-QPD X position" {
            w2406 = 2  # Channel pattern
            # "time average x2 the 3 psd signals (detection laser)"
            # "deinterlace 3 signals from qpds"
            n1005 = Decimate 1D Array(w2426) -> (w2425:i16[], w2424:i16[], w2407:i16[], w2423:i16[], w2369:i16[], w2366:i16[], w2363:i16[], w2394:i16[])
            n1006 = Select(t=i16 -1, s="Flip X Sign", f=i16 1) -> (s? t:f=w2359:i16)
            n1007 = Multiply(x=w2424, y=w2359) -> (x*y=w2360:i16[])
            n1008 = Decimate 1D Array(w2407) -> (w2392:i16[], w2390:i16[])
            n1009 = Decimate 1D Array(w2425) -> (w2422:i16[], w2409:i16[])
            n1010 = Decimate 1D Array(w2360) -> (w2421:i16[], w2419:i16[])
            n1011 = Decimate 1D Array(w2423) -> (w2420:i16[], w2418:i16[])
            n1012 = Decimate 1D Array(w2394) -> (w2393:i16[], w2391:i16[])
            n1013 = call "downsample 1D array - I16.vi"("Ave N"=2.0, "Array In"=w2369) -> ("Array Out"=w2367:i16[])  [unwired: 1 in]
            n1014 = call "downsample 1D array - I16.vi"("Ave N"=2.0, "Array In"=w2363) -> ("Array Out"=w2361:i16[])  [unwired: 1 in]
            n1015 = call "downsample 1D array - I16.vi"("Ave N"=2.0, "Array In"=w2366) -> ("Array Out"=w2364:i16[])  [unwired: 1 in]
            n1016 = Interleave 1D Arrays(w2422, w2421, w2420, w2409, w2419, w2418, w2393, w2392, w2391, w2390, w2367, w2364, w2361) -> (w2417:i16[])
            n1017 = Divide(x=w2417, y=3276.7) -> (x/y=w2416:dbl[])
            n1018 = Decimate 1D Array(w2416) -> (w2415:dbl[], w2414:dbl[], w2413:dbl[], w2412:dbl[], w2411:dbl[], w2410:dbl[], w2382:dbl[], w2380:dbl[], w2379:dbl[], w2377:dbl[], w2376:dbl[], w2375:dbl[], w2372:dbl[])
            n1019 = Negate(x=w2372) -> (-x=w2370:dbl[])
            n1020 = Divide(x=w2376, y=w2372) -> (x/y=w2374:dbl[])
            n1021 = Divide(x=w2375, y=w2370) -> (x/y=w2373:dbl[])
            n1022 = Divide(x=w2415, y=w2413) -> (x/y=w2398:dbl[])
            n1023 = Divide(x=w2414, y=w2413) -> (x/y=w2397:dbl[])
            n1024 = Divide(x=w2412, y=w2410) -> (x/y=w2396:dbl[])
            n1025 = Divide(x=w2411, y=w2410) -> (x/y=w2395:dbl[])
            n1026 = Divide(x=w2382, y=w2380) -> (x/y=w2381:dbl[])
            n1027 = Divide(x=w2379, y=w2377) -> (x/y=w2378:dbl[])
            n1028 = Build Array(w2398, w2397, w2413, w2396, w2395, w2410, w2381, w2380, w2378, w2377, w2374, w2373, w2372) -> (w2371:dbl[][])
            n1029 = Bundle("T1 Y", "T1 X", "T1 Sum", "T2 Y", "T2 X", "T2 Sum", "T1 FB X", "T1 FB Sum", "T2 FB X", "T2 FB Sum", "PSD Y", "PSD X", "PSD Y Sum") -> (w2399:T39)  [unwired: 1 out]
            n1030 = Cluster To Array(cluster=w2399) -> (array=w2408:string[])
          }
          frame "IR-QPD + PSD + FB-QPD XY positions" {
            w2473 = 4  # Channel pattern
            # "time average x2 the 3 psd signals (detection laser)"
            # "deinterlace 3 signals from qpds"
            n1031 = Decimate 1D Array(w2497) -> (w2496:i16[], w2495:i16[], w2474:i16[], w2494:i16[], w2440:i16[], w2486:i16[], w2485:i16[], w2462:i16[])
            n1032 = Decimate 1D Array "Feedback Sum"(w2474) -> (w2458:i16[], w2456:i16[])
            n1033 = Decimate 1D Array "QPD Y"(w2496) -> (w2493:i16[], w2476:i16[])
            n1034 = Decimate 1D Array "QPD X"(w2495) -> (w2492:i16[], w2490:i16[])
            n1035 = Decimate 1D Array "Feedback Y"(w2440) -> (w2439:i16[], w2438:i16[])
            n1036 = Decimate 1D Array "QPD Sum"(w2494) -> (w2491:i16[], w2489:i16[])
            n1037 = Decimate 1D Array "Feedback X"(w2462) -> (w2459:i16[], w2457:i16[])
            n1038 = call "downsample 1D array - double.vi"("Ave N"=2.0, "Array In"=w2486) -> ("Array Out"=w2461:dbl[])  [unwired: 1 out]
            n1039 = call "downsample 1D array - double.vi"("Ave N"=2.0, "Array In"=w2485) -> ("Array Out"=w2460:dbl[])  [unwired: 1 out]
            n1040 = Interleave 1D Arrays(w2493, w2492, w2491, w2476, w2490, w2489, w2439, w2459, w2458, w2438, w2457, w2456, w2461, w2460) -> (w2484:dbl[])
            n1041 = Divide(x=w2484, y=3276.7) -> (x/y=w2483:dbl[])
            n1042 = Decimate 1D Array(w2483) -> (w2482:dbl[], w2481:dbl[], w2480:dbl[], w2479:dbl[], w2478:dbl[], w2477:dbl[], w2435:dbl[], w2449:dbl[], w2433:dbl[], w2434:dbl[], w2447:dbl[], w2431:dbl[], w2445:dbl[], w2443:dbl[])
            n1043 = Negate(x=w2443) -> (-x=w2441:dbl[])
            n1044 = Divide(x=w2445, y=w2441) -> (x/y=w2444:dbl[])
            n1045 = Divide(x=w2434, y=w2431) -> (x/y=w2430:dbl[])
            n1046 = Divide(x=w2435, y=w2433) -> (x/y=w2432:dbl[])
            n1047 = Divide(x=w2482, y=w2480) -> (x/y=w2466:dbl[])
            n1048 = Divide(x=w2481, y=w2480) -> (x/y=w2465:dbl[])
            n1049 = Divide(x=w2479, y=w2477) -> (x/y=w2464:dbl[])
            n1050 = Divide(x=w2478, y=w2477) -> (x/y=w2463:dbl[])
            n1051 = Divide(x=w2449, y=w2433) -> (x/y=w2448:dbl[])
            n1052 = Divide(x=w2447, y=w2431) -> (x/y=w2446:dbl[])
            n1053 = Build Array(w2466, w2465, w2480, w2464, w2463, w2477, w2432, w2448, w2433, w2430, w2446, w2431, w2444, w2443) -> (w2442:dbl[][])
            n1054 = Bundle("T1 Y", "T1 X", "T1 Sum", "T2 Y", "T2 X", "T2 Sum", "T1 FB Y", "T1 FB X", "T1 FB Sum", "T2 FB Y", "T2 FB X", "T2 FB Sum", "PSD X", "PSD Y Sum") -> (w2429:T40)  [unwired: 1 out]
            n1055 = To Word Integer(number=w2484) -> (16bit integer=w2428:i16[])
            n1056 = Cluster To Array(cluster=w2429) -> (array=w2475:string[])
          }
        }
      }
    }
    "AI labels" <- w1557
    n1057 = Decimate 1D Array(w1531) -> (w1555:u32[], w1499:u32[])
    n1058 = local read "DMA Update Period (s)"() -> (w1567:dbl)
    n1059 = Build Array(w1555, w1499) -> (w1625:u32[][])
    n1060 = local read "Data Period (s)"() -> (w1405:dbl)
    n1061 = local read "BD 1 Frequency 2 (MHz)"() -> (w1438:dbl)
    n1062 = local read "BD 1 Frequency 1 (MHz)"() -> (w1439:dbl)
    n1063 = Decimate 1D Array(w1446) -> (w1470:i16[], w1469:i16[], w1467:i16[], w1466:i16[])  [unwired: 9 out]
    n1064 = To Double Precision Float(number=w1625) -> (double precision float=w1626:dbl[][])
    n1065 = local read "APD Integration Time (s)"() -> (w1512:dbl)
    n1066 = Multiply(x=w1405, y="Trap Pos. Disp. Downsample") -> (x*y=w1403:dbl)
    n1067 = Divide(x=w1470, y=w1469) -> (x/y=w1471:dbl[])
    n1068 = Divide(x=w1467, y=w1466) -> (x/y=w1468:dbl[])
    n1069 = feedback #6(0.0) -> (w1484:dbl)
    n1070 = Add(x=w1567, y=w1484) -> (x+y=w1665:dbl)
    n1071 = feedback-in #6(w1665) -> ()
    n1072 = local read "AOM X Cal (nm/MHz)"() -> (w1436:dbl)
    n1073 = To Time Stamp(1:w1484) -> (0:w1483:timestamp)
    n1074 = Split 1D Array(array=w1471, index="N El. to Ave.") -> (second subarray=w1474:dbl[])  [unwired: 1 out]
    n1075 = Split 1D Array(array=w1468, index="N El. to Ave.") -> (second subarray=w1473:dbl[])  [unwired: 1 out]
    n1076 = Multiply(x=w1405, y="Trap Disp. Downsample") -> (x*y=w1485:dbl)
    "Display Period (s)" <- w1485
    n1077 = for "Trap AI" {
      tunnel: [w2222] -> w1659 mode=indexing
      tunnel: w1483 -> [w2212]
      tunnel: "Trap Disp. Downsample" -> [w2220]
      tunnel: w1558 -> [w2218] mode=indexing
      tunnel: w1405 -> [w2217]
      tunnel: w1557 -> [w2216] mode=indexing
      tunnel: w1482 -> [w2215]
